vi "SlowModeRamping.vi"(9 "Ramp Time (ms)":u32=10000, 10 "Goal":i32=25, 11 "SlowMode?":bool) -> (3 "Multiplier":dbl)   [LabVIEW 2013]
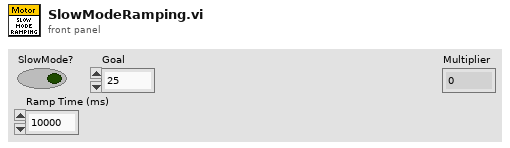
[diagram p1: front panel]
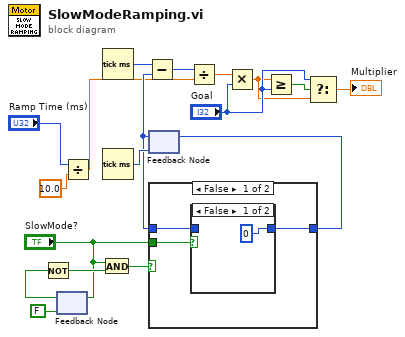
[diagram p0: block diagram]
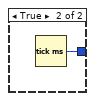
[diagram p3: hidden frame]
diagram:
  n1 = feedback-in #1("SlowMode?") -> ()
  n2 = feedback #1(FALSE ("Boolean")) -> (w16:bool)
  n3 = Not(x=w16) -> (.not. x?=w18:bool)
  n4 = Divide(x="Ramp Time (ms)", y=10.0) -> (x/y=w3:dbl)
  n5 = And(x="SlowMode?", y=w18) -> (x .and. y?=w15:bool)
  n6 = Tick Count (ms)() -> (millisecond timer value=w10:u32)
  n7 = Tick Count (ms)() -> (millisecond timer value=w13:u32)
  n8 = feedback #2(w13) -> (w9:u32)
  n9 = Subtract(x=w10, y=w9) -> (x-y=w12:u32)
  n10 = case shown="False" w15 {
    tunnel: [w21 w24] -> w14
    tunnel: w9 -> [w20 _]
    tunnel: "SlowMode?" -> [w19 _]
    frame False {
      n11 = case shown="False" w19 {
        tunnel: [u32 0 ("millisecond timer value") w23] -> w21
        tunnel: w20 -> [_ w23]
        frame False {
        }
        frame True {
        }
      }
    }
    frame True {
      n12 = Tick Count (ms)() -> (millisecond timer value=w24:u32)
    }
  }
  n13 = feedback-in #2(w14) -> ()
  n14 = Divide(x=w12, y=w3) -> (x/y=w11:dbl)
  n15 = Multiply(x=w11, y="Goal") -> (x*y=w6:dbl)
  n16 = Greater Or Equal?(x=w6, y="Goal") -> (x >= y?=w8:bool)
  n17 = Select(t="Goal", s=w8, f=w6) -> (s? t:f=→"Multiplier":dbl)
